vi "Send Message.vi"(8 "error in (no error)":errorcluster, 10 "Message Data":string, 11 "Web Client in":refnum<class "Web Client.lvclass">) -> (0 "error out":errorcluster, 2 "Response":string, 3 "Web Client out":refnum<class "Web Client.lvclass">)   [LabVIEW 2018, in "Collaborator.lvlib" / "Web Client.lvclass"]
uses:
  Web Client.lvclass
  Web Client.lvclass/Web Client.ctl
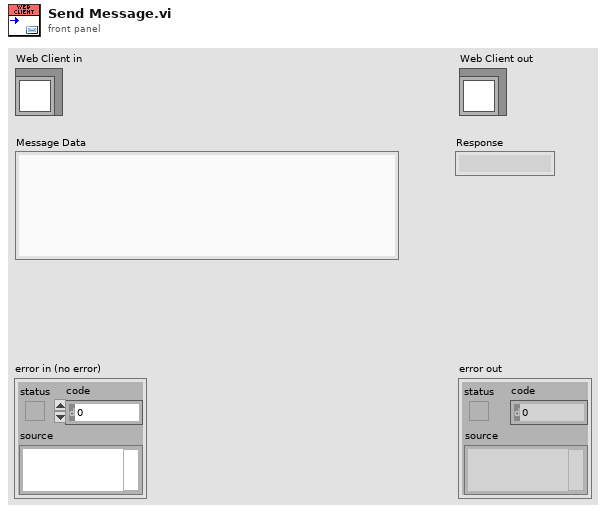
[diagram p1: front panel]
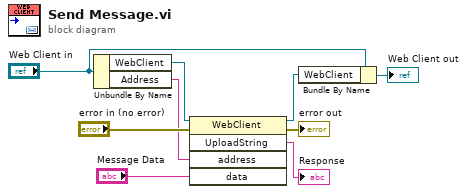
[diagram p0: block diagram]
diagram:
  n1 = Unbundle By Name("Web Client in") -> ("WebClient"=w5:refnum<k24>, "Address"=w3:string)
  n2 = invoke class="WebClient" method="UploadString"(reference=w5, error in="error in (no error)", "address"=w3, "data"="Message Data") -> (reference out=w4:refnum<k24>, error out=→"error out":errorcluster, "UploadString"=→"Response":string)  [unwired: 1 in, 2 out]
  n3 = Bundle By Name(cluster="Web Client in", "WebClient"=w4) -> (→"Web Client out":refnum<class "Web Client.lvclass">)
